vi "PartInfo.vi"(5 "OP":string, 6 "Time":string, 7 "Date Code":string, 8 "W/O":string, 9 "model":string, 10 "Lot#":string, 11 "P/N":string) -> (0 "output string":string)   [LabVIEW 2013]
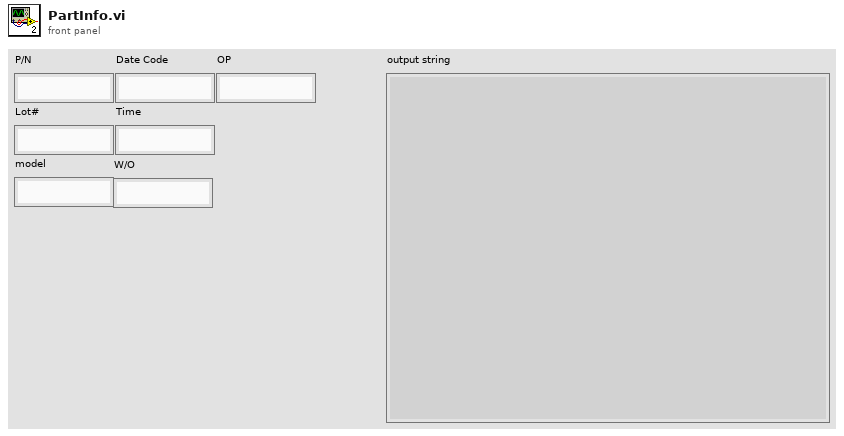
[diagram p1: front panel]
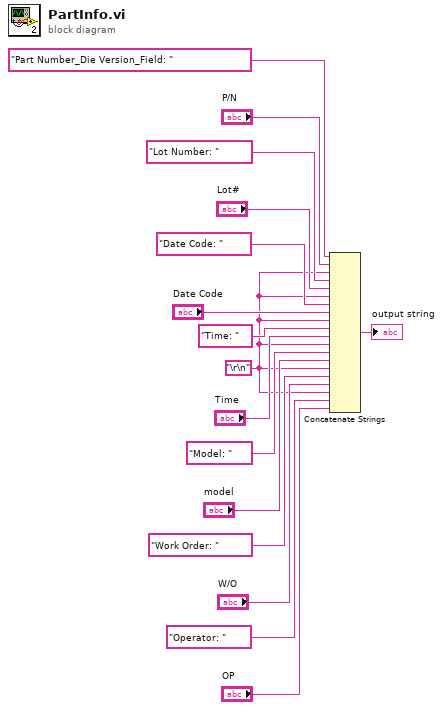
[diagram p0: block diagram]
diagram:
  w3 = "\r\n"
  n1 = Concatenate Strings("Part Number_Die Version_Field: " ("string"), "P/N", w3, "Lot Number: " ("string"), "Lot#", w3, "Date Code: " ("string"), "Date Code", w3, "Time: " ("string"), "Time", w3, "Model: " ("string"), "model", w3, "Work Order: " ("string"), "W/O", w3, "Operator: " ("string"), "OP") -> (→"output string":string)
